vi "Graphical Solution to alpha_n.vi"(6 "Quantum Number":i32=1, 8 "error in":errorcluster, 11 "R":dbl=7.0) -> (0 "error out":errorcluster, 2 "XY Graph":cluster{"x":dbl[], "y":dbl[]}[](graph), 3 "alpha_n":dbl[](array[numeric]))   [LabVIEW 2023]
doc: "When attempting to solve Schrodinger's equation for when a particle is trapped in a finite potential well, a system of equations is encountered that cannot be solved analytically. This VI shows how to solve them numerically."
panel:
  # "Note: This is a subVI used by the Finite Potential Well.vi example. The instructions below allow you to experiment with the effect of the R value on the solution.\n\n1. Run this VI continuously.\n2. You will get the solutions to the  system of equations shown on left  top corner of the front panel as red dots on the graph.\n3. Play with the value of R. Increase or decrease it. You will see the green circle graph move and recalculate the new solutions."
  # "Find solutions (alpha_n) of the two equations graphically"
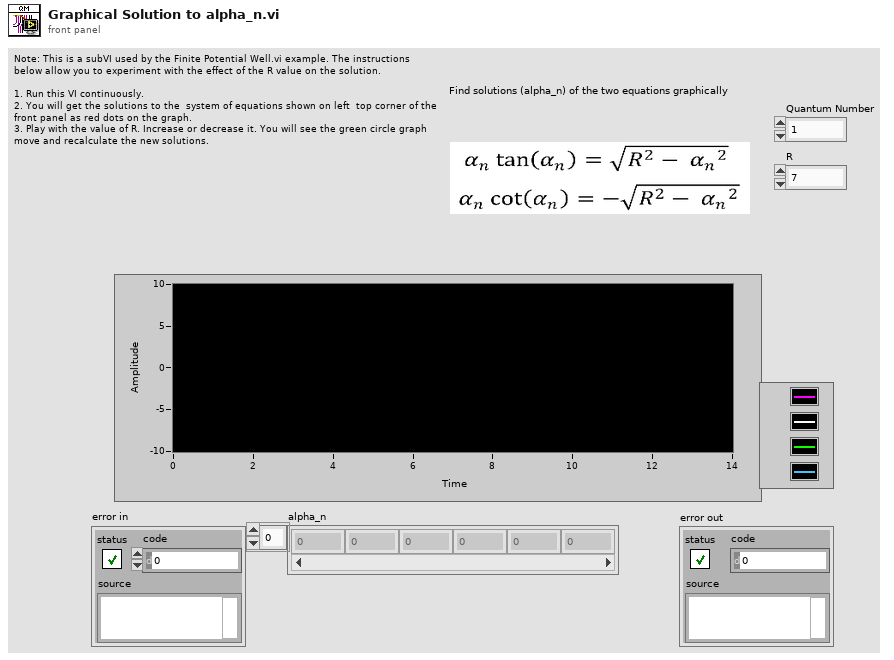
[diagram p1: front panel]
types:
  T1 = cluster{"plots":cluster{"x":dbl[], "y":dbl[]}[], "xs":dbl[]}
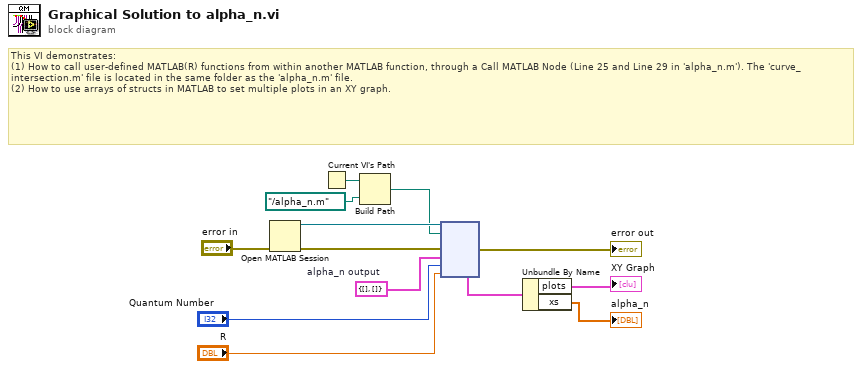
[diagram p0: block diagram]
diagram:
  w1 = T1 {"plots"=[], "xs"=[]}  # alpha_n output
  # "This VI demonstrates:\n(1) How to call user-defined MATLAB(R) functions from within another MATLAB function, through a Call MATLAB Node (Line 25 and Line 29 in 'alpha_n.m'). The 'curve_intersection.m' file is located in the same folder as the 'alpha_n.m' file.\n(2) How to use arrays of structs in MATLAB to set multiple plots in an XY graph."
  n1 = Open MATLAB Session(3:"error in") -> (8:w13:refnum<k37>, 11:w12:errorcluster)  [unwired: 1 in]
  n2 = Current VI's Path() -> (path=w11:path)
  n3 = Build Path(base path=w11, name or relative path=path "../alpha_n.m") -> (appended path=w9:path)
  n4 = node(w13, w9, w12, w1, "Quantum Number", "R") -> (→"error out":errorcluster, w6:T1)  [unwired: 3 in, 3 out]
  n5 = Unbundle By Name(w6) -> ("plots"=→"XY Graph":cluster{"x":dbl[], "y":dbl[]}[], "xs"=→"alpha_n":dbl[])
